vi "Team Editor and Schedule Creator.vi"(8 "Edit?":bool=TRUE, 11 "TeamData_and_Schedule IN":T2) -> (0 "LegacyTeamInfo":T1, 1 "RAW Schedule":string[][](array[string]), 2 "String Schedule":string[][](array[string]), 3 "TeamData_and_Schedule OUT":T2, 4 "MatchEqualizationString":string[][](array[string]), 5 "Cancelled?":bool=TRUE, 6 "MatchEqualizationInteger":i32[](array[numeric]))   [LabVIEW 2013]
uses:
  Team Data Array2.ctl
  TeamData_and_Schedule.ctl
  Legacy_Team_Info.ctl
  <vilib>/Utility/sysdir.llb/System Directory Type.ctl
  <vilib>/Utility/xml.llb/Write to XML File(string).vi
  <vilib>/Utility/xml.llb/Read From XML File(string).vi
panel:
  out "Team Number Schedule":i32[][](array[numeric])
  out "Match Array (indices)":i32[][](array[numeric])
  out "NextState":i32
  in  "Team Info":T3
  in  "Tab Control":T4(tab)
  out "String":string="NOTE:  You are not allowed to Add or Delete teams once you've started submitting scores for teams.  Doing so may drop scores, or assign scores to the wrong teams!\n\nOnce you've begun submitting scores, you are only allowed to edit the team information."
  in  "Load Team List Button":bool
  in  "Save Team List Button":bool
  in  "Number of Teams:":dbl
  in  "Cancel Button":bool
  in  "OK Button":bool
  in  "Edit Team Button":bool
  in  "Remove Team Button":bool
  in  "Add Team Button":bool
  in  "Competing Team List":i32(listbox)
  in  "Add Team Back Button":bool
  in  "Add Team Next Button":bool
  out "Add Team String":string="Add a Team\n\nEnter Team Information and press NEXT.  To cancel, press BACK.  You are required to provide a TEAM NUMBER greater than ZERO and a non-blank Team Name."
  in  "Team Number":dbl
  in  "Team Name":string
  in  "Remove Team Back Button":bool
  in  "Remove Team Next Button":bool
  out "Remove Team String":string="Remove a Team\n\nSelect Team to Remove and press NEXT.  To cancel, press BACK.  If you press NEXT, the selected team will be removed."
  in  "Team To Remove":u16(ring)
  in  "Edit Team Back Button":bool
  in  "Edit Team Next Button":bool
  out "Rename Team String":string="Rename a Team\n\nSelect a Team to be Renamed, then type in the NEW name of the team in the \"New Team Name\" field.  The New Team Name cannot be blank. Press NEXT to rename the team, or BACK to cancel."
  in  "Team to Edit":u16(ring) items=["10, Team One Oh"=0, "20, Twenty is Plenty"=1, "40, The Shorty Forty "=3, "42, The Ultimate Answer"=4, "50, Half Century Team"=5, "60, The Golden Years"=6, "70, One Plus LASA Robotics"=7, "80, Eighty is Greaty"=8, "90, Ten to a Century"=9, "100, Century Mark Team"=10]
  in  "New Team Name":string
  in  "New Team Number":dbl
  out "Error String":string
  in  "Error Back Button":bool
  in  "Back-To-Back Interval":dbl=1.0 min=0.0 max=8.0 step=1.0
  in  "Matches per Team":dbl=1.0 min=1.0 max=10.0 step=1.0
  in  "Number of Fields":dbl=1.0 min=1.0 max=2.0 step=1.0
  out "Create Schedule String":string="Create Schedule\n\nEnter the required information below.  \n\nNumber of Fields - Number of fields you have.  A field is composed of 4 quadrants that play simultaneously.\n\nMatches per Team - Number of matches each team is to be scheduled to play during the competition.\n\nBack-To-Back Interval - Minimum number of matches that can take place between when a team plays and when they have to play next."
  in  "CreateSched Back Button":bool
  in  "CreateSched Next Button":bool
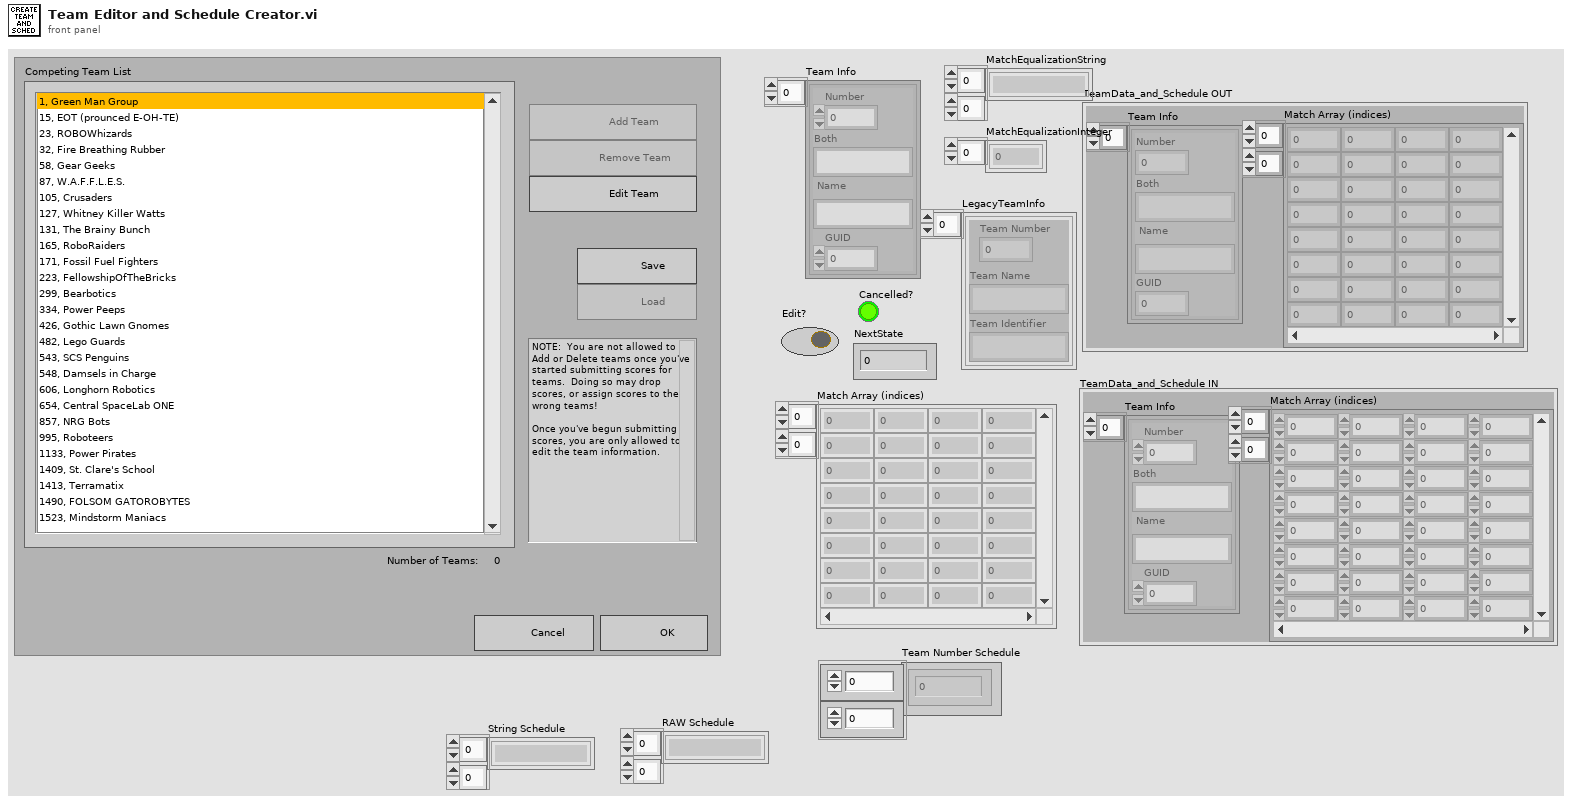
[diagram p1: front panel]
types:
  T1 = typedef "Legacy_Team_Info.ctl" = cluster{"Team Number":i32, "Team Name":string, "Team Identifier":string}[]
  T2 = typedef "TeamData_and_Schedule.ctl" = cluster{"Team Info":cluster{"Number":u16, "Both":string, "Name":string, "GUID":u16}[], "Match Array (indices)":i32[][]}
  T3 = typedef "Team Data Array2.ctl" = cluster{"Number":u16, "Both":string, "Name":string, "GUID":u16}[]
  T4 = enum32{"Main Page", "Add Team", "Remove Team", "Rename Team", "Errors", "Schedule"}
  T5 = enum8{"Enabled", "Disabled", "Disabled and Grayed Out"}
  T6 = cluster{"Number":u16, "Both":string, "Name":string, "GUID":u16}[]
  T7 = enum32{"Main Page", "Add Team", "Remove Team", "Rename Team", "Errors"}
  T8 = typedef "System Directory Type.ctl" = i32
  T9 = typedef "LVStringsAndValuesArrayTypeDef_U16.ctl" = cluster{"String":string, "Value":u16}[]
  T10 = cluster{"Team Number":i32, "Team Name":string, "Team Identifier":string}
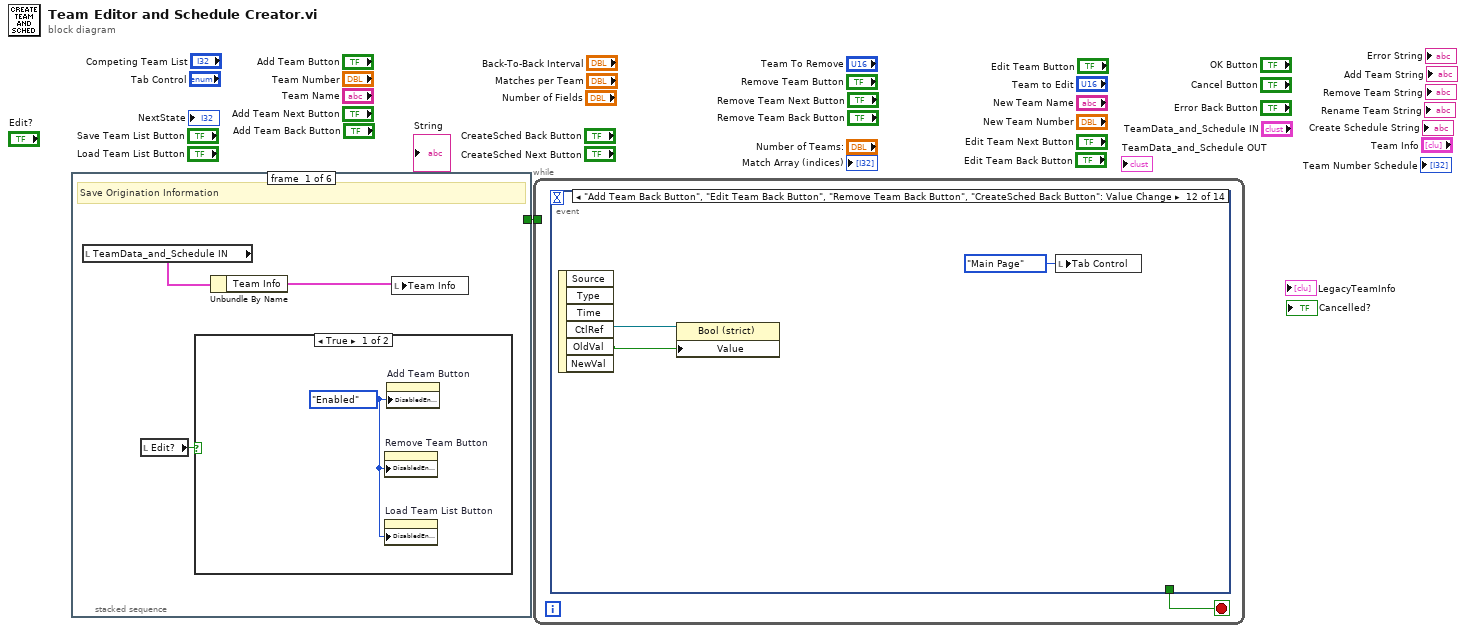
[diagram p0: block diagram]
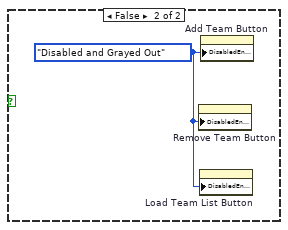
[diagram p2: hidden frame]
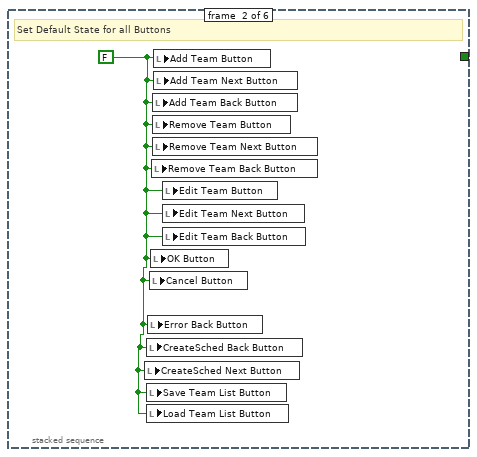
[diagram p3: hidden frame]
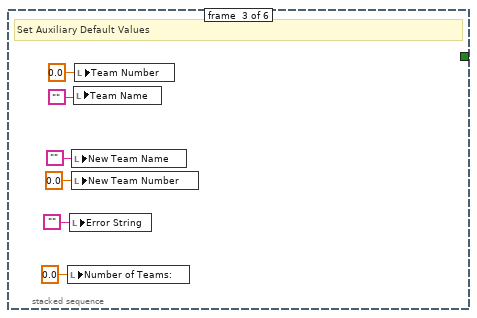
[diagram p4: hidden frame]
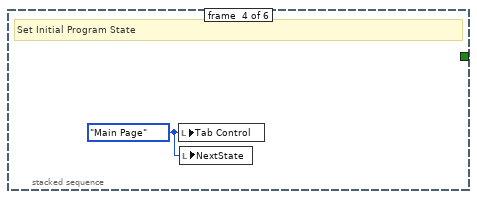
[diagram p5: hidden frame]
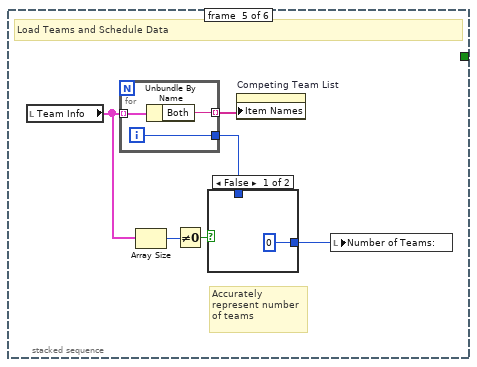
[diagram p6: hidden frame]
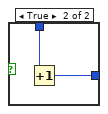
[diagram p7: hidden frame]
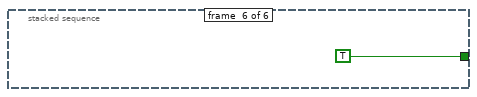
[diagram p8: hidden frame]
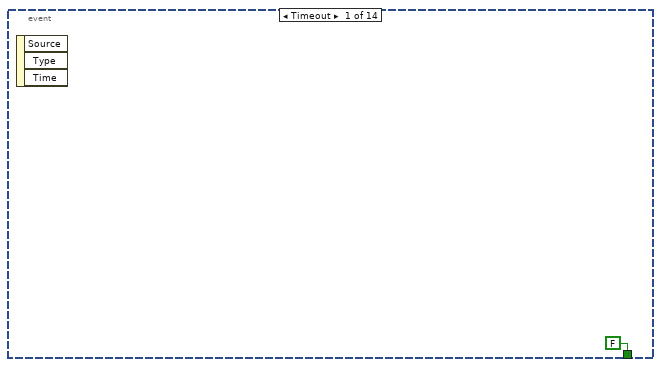
[diagram p9: hidden frame]
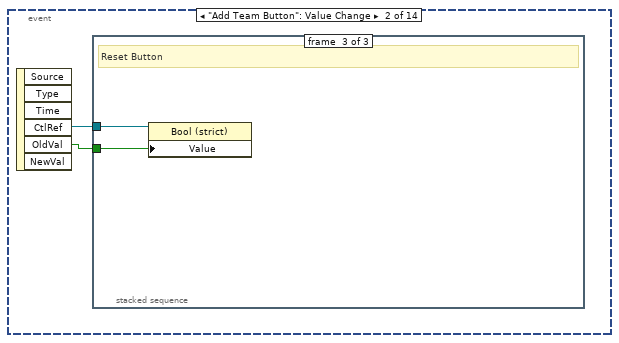
[diagram p10: hidden frame]
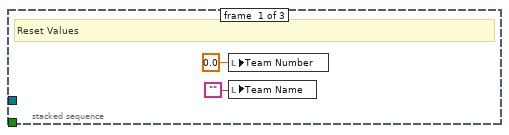
[diagram p11: hidden frame]
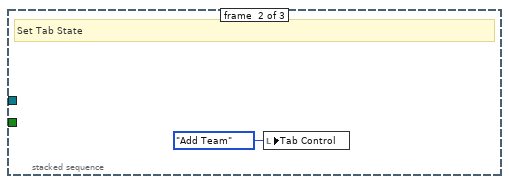
[diagram p12: hidden frame]
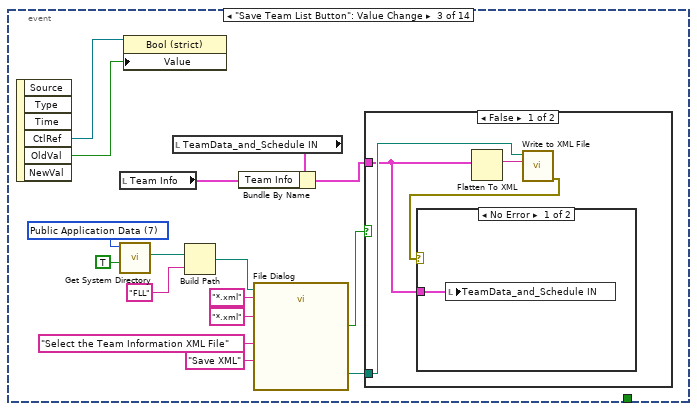
[diagram p13: hidden frame]
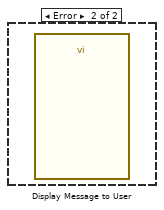
[diagram p14: hidden frame]
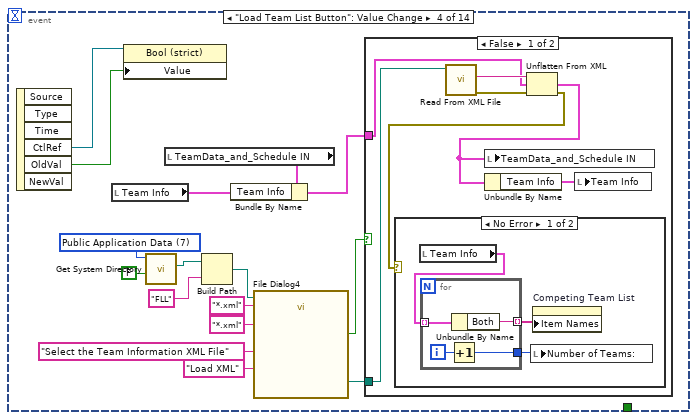
[diagram p16: hidden frame]
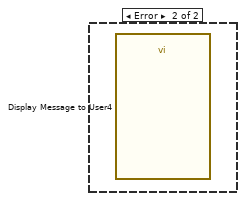
[diagram p17: hidden frame]
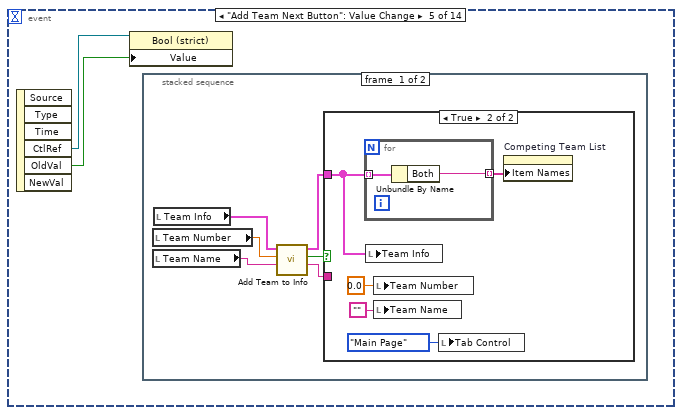
[diagram p19: hidden frame]
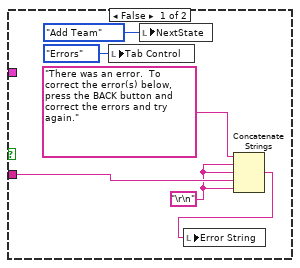
[diagram p20: hidden frame]
diagram:
  n1 = stacked-sequence {
    tunnel: [_ _ _ _ _ TRUE] -> w1
    frame #0 {
      # "Save Origination Information"
      n2 = local read "TeamData_and_Schedule IN"() -> (w4:T2)
      n3 = local read "Edit?"() -> (w2:bool)
      n4 = case shown="True" w2 {
        frame True {
          w5 = T5."Enabled" ("Disabled")
          n5 = property on="Remove Team Button" class="Bool (strict)"("DisabledEnum"=w5) -> ()  [unwired: 2 in, 2 out]
          n6 = property on="Load Team List Button" class="Bool (strict)"("DisabledEnum"=w5) -> ()  [unwired: 2 in, 2 out]
          n7 = property on="Add Team Button" class="Bool (strict)"("DisabledEnum"=w5) -> ()  [unwired: 2 in, 2 out]
        }
        frame False {
          w6 = T5."Disabled and Grayed Out" ("Disabled")
          n8 = property on="Remove Team Button" class="Bool (strict)"("DisabledEnum"=w6) -> ()  [unwired: 2 in, 2 out]
          n9 = property on="Load Team List Button" class="Bool (strict)"("DisabledEnum"=w6) -> ()  [unwired: 2 in, 2 out]
          n10 = property on="Add Team Button" class="Bool (strict)"("DisabledEnum"=w6) -> ()  [unwired: 2 in, 2 out]
        }
      }
      n11 = Unbundle By Name(w4) -> ("Team Info"=w3:T6)
      n12 = local write "Team Info"(w3) -> ()
    }
    frame #1 {
      w7 = FALSE
      # "Set Default State for all Buttons"
      n13 = local write "CreateSched Next Button"(w7) -> ()
      n14 = local write "CreateSched Back Button"(w7) -> ()
      n15 = local write "Save Team List Button"(w7) -> ()
      n16 = local write "Load Team List Button"(w7) -> ()
      n17 = local write "Error Back Button"(w7) -> ()
      n18 = local write "Cancel Button"(w7) -> ()
      n19 = local write "OK Button"(w7) -> ()
      n20 = local write "Remove Team Back Button"(w7) -> ()
      n21 = local write "Add Team Back Button"(w7) -> ()
      n22 = local write "Remove Team Button"(w7) -> ()
      n23 = local write "Remove Team Next Button"(w7) -> ()
      n24 = local write "Add Team Button"(w7) -> ()
      n25 = local write "Add Team Next Button"(w7) -> ()
      n26 = local write "Edit Team Button"(w7) -> ()
      n27 = local write "Edit Team Next Button"(w7) -> ()
      n28 = local write "Edit Team Back Button"(w7) -> ()
    }
    frame #2 {
      # "Set Auxiliary Default Values"
      n29 = local write "Number of Teams:"(0.0 ("Number of Teams:")) -> ()
      n30 = local write "Error String"("") -> ()
      n31 = local write "New Team Name"("") -> ()
      n32 = local write "New Team Number"(0.0 ("New Team Number")) -> ()
      n33 = local write "Team Name"("") -> ()
      n34 = local write "Team Number"(0.0 ("Team Number")) -> ()
    }
    frame #3 {
      w14 = T7."Main Page" ("Tab Control")
      # "Set Initial Program State"
      n35 = local write "Tab Control"(w14) -> ()
      n36 = local write "NextState"(w14) -> ()
    }
    frame #4 {
      # "Accurately \nrepresent number\nof teams"
      # "Load Teams and Schedule Data"
      n37 = local read "Team Info"() -> (w17:T3)
      n38 = for {
        tunnel: w17 -> [w26] mode=indexing
        tunnel: [w25] -> w20 mode=indexing
        tunnel: [w24] -> w19
        i -> [w24]
        n39 = Unbundle By Name(w26) -> ("Both"=w25:string)
      }
      n40 = Array Size(array=w17) -> (size(s)=w16:i32)
      n41 = Not Equal To 0?(x=w16) -> (x != 0?=w15:bool)
      n42 = case shown="False" w15 {
        tunnel: w19 -> [_ w23]
        tunnel: [0 w22] -> w18
        frame False {
        }
        frame True {
          n43 = Increment(x=w23) -> (x+1=w22:i32)
        }
      }
      n44 = property on="Competing Team List" class="LstBox (strict)"("Item Names"=w20) -> ()  [unwired: 2 in, 2 out]
      n45 = local write "Number of Teams:"(w18) -> ()
    }
    frame #5 {
    }
  }
  n46 = while {
    tunnel: w1 -> [_]
    stop <- w28 stop-if-true
    n47 = event shown="[11] \"Add Team Back Button\", \"Edit Team Back Button\", \"Remove Team Back Button\", \"CreateSched Back Button\": Value Change" {
      selector: _ -> [_ _ _ _ _ _ _ _ _ _ _ _ _ _]
      dyn-events: _ -> [_ _ _ _ _ _ _ _ _ _ _ _ _ _]
      timeout: _ -> [_ _ _ _ _ _ _ _ _ _ _ _ _ _]
      tunnel: [FALSE _ _ _ _ _ _ _ _ _ _ _ TRUE TRUE] -> w28
      event Timeout {
        n48 = event-data() -> ()  [unwired: 1 in, 3 out]
      }
      event "Add Team Button": Value Change {
        n49 = event-data() -> ("CtlRef"=w31:refnum<vi>, "OldVal"=w30:bool)  [unwired: 1 in, 4 out]
        n50 = stacked-sequence {
          tunnel: w31 -> [_ _ w36]
          tunnel: w30 -> [_ _ w35]
          frame #0 {
            # "Reset Values"
            n51 = local write "Team Number"(0.0 ("Team Number")) -> ()
            n52 = local write "Team Name"("") -> ()
          }
          frame #1 {
            # "Set Tab State"
            n53 = local write "Tab Control"(T7."Add Team" ("Tab Control")) -> ()
          }
          frame #2 {
            # "Reset Button"
            n54 = property class="Bool (strict)"(reference=w36, "Value"=w35) -> ()  [unwired: 1 in, 2 out]
          }
        }
      }
      event "Save Team List Button": Value Change {
        w44 = T8 7 items=["User Home"=0, "User Desktop"=1, "User Documents"=2, "User Application Data"=3, "User Preferences"=4, "User Temporary"=5, "Public Documents"=6, "Public Application Data"=7, "Public Preferences"=8, "Public Cache"=13, "System Core Libraries"=9, "System Installed Libraries"=10, "Application Files"=11, "Boot Volume Root"=12] ("system directory type")
        n55 = event-data() -> ("CtlRef"=w52:refnum<vi>, "OldVal"=w51:bool)  [unwired: 1 in, 4 out]
        n56 = local read "Team Info"() -> (w41:T3)
        n57 = call <vilib>:"Get System Directory.vi"("create directory if not found? (F)"=TRUE, "system directory type"=w44) -> ("system directory"=w39:path)  [unwired: 9 in]
        n58 = property class="Bool (strict)"(reference=w52, "Value"=w51) -> ()  [unwired: 1 in, 2 out]
        n59 = local read "TeamData_and_Schedule IN"() -> (w42:T2)
        n60 = Build Path(base path=w39, name or relative path="FLL") -> (appended path=w37:path)
        n61 = Bundle By Name(cluster=w42, "Team Info"=w41) -> (w40:T2)
        n62 = call "File Dialog"("start path"=w37, "prompt"="Select the Team Information XML File", "button label"="Save XML", "pattern (all files)"="*.xml", "pattern label"="*.xml") -> ("selected path"=w45:path, "cancelled"=w46:bool)  [unwired: 7 in, 2 out]
        n63 = case shown="False" w46 {
          tunnel: w45 -> [w55 _]
          tunnel: w40 -> [w53 _]
          frame False {
            n64 = Flatten To XML(anything=w53) -> (xml string=w56:string)
            n65 = call-poly <vilib>:"Write to XML File.vi"("XML Input"=w56, "XML File Path"=w55) -> ("error out"=w54:errorcluster)  [unwired: 7 in, 2 out]
            n66 = case shown="No Error" w54 {
              tunnel: w53 -> [w57 _]
              frame No Error {
                n67 = local write "TeamData_and_Schedule IN"(w57) -> ()
              }
              frame Error {
                n68 = call "Display Message to User"() -> ()  [unwired: 10 in, 2 out]
              }
            }
          }
          frame True {
          }
        }
      }
      event "Load Team List Button": Value Change {
        w65 = T8 7 items=["User Home"=0, "User Desktop"=1, "User Documents"=2, "User Application Data"=3, "User Preferences"=4, "User Temporary"=5, "Public Documents"=6, "Public Application Data"=7, "Public Preferences"=8, "Public Cache"=13, "System Core Libraries"=9, "System Installed Libraries"=10, "Application Files"=11, "Boot Volume Root"=12] ("system directory type")
        n69 = event-data() -> ("CtlRef"=w73:refnum<vi>, "OldVal"=w72:bool)  [unwired: 1 in, 4 out]
        n70 = local read "Team Info"() -> (w62:T3)
        n71 = property class="Bool (strict)"(reference=w73, "Value"=w72) -> ()  [unwired: 1 in, 2 out]
        n72 = call <vilib>:"Get System Directory.vi"("create directory if not found? (F)"=FALSE, "system directory type"=w65) -> ("system directory"=w60:path)  [unwired: 9 in]
        n73 = local read "TeamData_and_Schedule IN"() -> (w63:T2)
        n74 = Build Path(base path=w60, name or relative path="FLL") -> (appended path=w58:path)
        n75 = Bundle By Name(cluster=w63, "Team Info"=w62) -> (w61:T2)
        n76 = call "File Dialog4"("start path"=w58, "prompt"="Select the Team Information XML File", "button label"="Load XML", "pattern (all files)"="*.xml", "pattern label"="*.xml") -> ("selected path"=w66:path, "cancelled"=w67:bool)  [unwired: 7 in, 2 out]
        n77 = case shown="False" w67 {
          tunnel: w66 -> [w80 _]
          tunnel: w61 -> [w78 _]
          frame False {
            n78 = call-poly <vilib>:"Read From XML File.vi"("XML File Path"=w80) -> ("error out"=w76:errorcluster, "XML Elements"=w79:string)  [unwired: 8 in, 1 out]
            n79 = Unflatten From XML(xml string=w79, type=w78, error in (no error)=w76) -> (value=w74:T2, error out=w77:errorcluster)
            n80 = case shown="No Error" w77 {
              frame No Error {
                n81 = local read "Team Info"() -> (w83:T3)
                n82 = for {
                  tunnel: w83 -> [w87] mode=indexing
                  tunnel: [w86] -> w82 mode=indexing
                  tunnel: [w84] -> w81
                  i -> [w85]
                  n83 = Increment(x=w85) -> (x+1=w84:i32)
                  n84 = Unbundle By Name(w87) -> ("Both"=w86:string)
                }
                n85 = local write "Number of Teams:"(w81) -> ()
                n86 = property on="Competing Team List" class="LstBox (strict)"("Item Names"=w82) -> ()  [unwired: 2 in, 2 out]
              }
              frame Error {
                n87 = call "Display Message to User4"() -> ()  [unwired: 10 in, 2 out]
              }
            }
            n88 = local write "TeamData_and_Schedule IN"(w74) -> ()
            n89 = Unbundle By Name(w74) -> ("Team Info"=w75:T6)
            n90 = local write "Team Info"(w75) -> ()
          }
          frame True {
          }
        }
      }
      event "Add Team Next Button": Value Change {
        n91 = event-data() -> ("CtlRef"=w89:refnum<vi>, "OldVal"=w88:bool)  [unwired: 1 in, 4 out]
        n92 = property class="Bool (strict)"(reference=w89, "Value"=w88) -> ()  [unwired: 1 in, 2 out]
        n93 = stacked-sequence {
          frame #0 {
            n94 = local read "Team Number"() -> (w94:dbl)
            n95 = local read "Team Name"() -> (w95:string)
            n96 = local read "Team Info"() -> (w93:T3)
            n97 = call "Add Team to Info.vi"("Team Name"=w95, "Team Number"=w94, "Team Info in"=w93) -> ("Error String"=w90:string, "Team Added?"=w92:bool, "Team Info out"=w91:T3)  [unwired: 6 in]
            n98 = case shown="True" w92 {
              tunnel: w91 -> [_ w104]
              tunnel: w90 -> [w99 _]
              frame False {
                w98 = "\r\n"
                n99 = local write "Tab Control"(T7."Errors" ("Tab Control")) -> ()
                n100 = local write "NextState"(T7."Add Team" ("Tab Control")) -> ()
                n101 = Concatenate Strings("There was an error.  To correct the error(s) below, press the BACK button and correct the errors and try again.", w98, w98, w99, w98) -> (w97:string)
                n102 = local write "Error String"(w97) -> ()
              }
              frame True {
                n103 = for {
                  tunnel: w104 -> [w108] mode=indexing
                  tunnel: [w107] -> w106 mode=indexing
                  n104 = Unbundle By Name(w108) -> ("Both"=w107:string)
                }
                n105 = local write "Team Info"(w104) -> ()
                n106 = local write "Team Number"(0.0 ("Team Number")) -> ()
                n107 = local write "Team Name"("") -> ()
                n108 = local write "Tab Control"(T7."Main Page" ("Tab Control")) -> ()
                n109 = property on="Competing Team List" class="LstBox (strict)"("Item Names"=w106) -> ()  [unwired: 2 in, 2 out]
              }
            }
          }
          frame #1 {
            n110 = property on="Competing Team List" class="LstBox (strict)"() -> ("Item Names"=w110:string[])  [unwired: 2 in, 2 out]
            n111 = Array Size(array=w110) -> (size(s)=w109:i32)
            n112 = local write "Number of Teams:"(w109) -> ()
          }
        }
      }
      event "Edit Team Next Button": Value Change {
        n113 = event-data() -> ("CtlRef"=w112:refnum<vi>, "OldVal"=w111:bool)  [unwired: 1 in, 4 out]
        n114 = stacked-sequence {
          frame #0 {
            n115 = local read "New Team Number"() -> (w118:dbl)
            n116 = local read "New Team Name"() -> (w119:string)
            n117 = local read "Team to Edit"() -> (w113:u16)
            n118 = local read "Team Info"() -> (w117:T3)
            n119 = call "Edit Team in Info.vi"("Team GUID"=w113, "New Team Name"=w119, "New Team Number"=w118, "Team Info in"=w117) -> ("Error String"=w114:string, "Team Edited?"=w116:bool, "Team Info out"=w115:T3)  [unwired: 5 in]
            n120 = case shown="False" w116 {
              tunnel: w115 -> [_ w128]
              tunnel: w114 -> [w123 _]
              frame False {
                w122 = "\r\n"
                n121 = local write "Tab Control"(T7."Errors" ("Tab Control")) -> ()
                n122 = local write "NextState"(T7."Rename Team" ("Tab Control")) -> ()
                n123 = Concatenate Strings("There was an error.  To correct the error(s) below, press the BACK button and correct the errors and try again.", w122, w122, w123, w122) -> (w121:string)
                n124 = local write "Error String"(w121) -> ()
              }
              frame True {
                n125 = for {
                  tunnel: w128 -> [w132] mode=indexing
                  tunnel: [w131] -> w130 mode=indexing
                  n126 = Unbundle By Name(w132) -> ("Both"=w131:string)
                }
                n127 = local write "Team Info"(w128) -> ()
                n128 = local write "New Team Number"(0.0 ("Team Number")) -> ()
                n129 = local write "New Team Name"("") -> ()
                n130 = local write "Tab Control"(T7."Main Page" ("Tab Control")) -> ()
                n131 = property on="Competing Team List" class="LstBox (strict)"("Item Names"=w130) -> ()  [unwired: 2 in, 2 out]
              }
            }
          }
          frame #1 {
            n132 = property on="Competing Team List" class="LstBox (strict)"() -> ("Item Names"=w134:string[])  [unwired: 2 in, 2 out]
            n133 = Array Size(array=w134) -> (size(s)=w133:i32)
            n134 = local write "Number of Teams:"(w133) -> ()
          }
        }
        n135 = property class="Bool (strict)"(reference=w112, "Value"=w111) -> ()  [unwired: 1 in, 2 out]
      }
      event "Error Back Button": Value Change {
        n136 = event-data() -> ("CtlRef"=w136:refnum<vi>, "OldVal"=w135:bool)  [unwired: 1 in, 4 out]
        n137 = property class="Bool (strict)"(reference=w136, "Value"=w135) -> ()  [unwired: 1 in, 2 out]
        n138 = local read "NextState"() -> (w137:i32)
        n139 = local write "Tab Control"(w137) -> ()
      }
      event "Remove Team Button": Value Change {
        n140 = event-data() -> ("CtlRef"=w139:refnum<vi>, "OldVal"=w138:bool)  [unwired: 1 in, 4 out]
        n141 = stacked-sequence {
          tunnel: w139 -> [_ _ w155]
          tunnel: w138 -> [_ _ w154]
          frame #0 {
            # "Reset Values"
            n142 = stacked-sequence {
              frame #0 {
                n143 = local read "Team Info"() -> (w141:T3)
                n144 = for {
                  tunnel: w141 -> [w145] mode=indexing
                  tunnel: [w142] -> w140 mode=indexing
                  n145 = Unbundle By Name(w145) -> ("Both"=w143:string, "GUID"=w144:u16)
                  n146 = Bundle("Both"=w143, "GUID"=w144) -> (w142:cluster{"Both":string, "GUID":u16})  [unwired: 1 in]
                }
                n147 = property on="Team To Remove" class="Ring (strict)"("StringsAndValues[]"=w140) -> ()  [unwired: 2 in, 2 out]
              }
              frame #1 {
                n148 = local read "Competing Team List"() -> (w149:i32)
                n149 = property on="Team To Remove" class="Ring (strict)"() -> ("StringsAndValues[]"=w152:T9)  [unwired: 2 in, 2 out]
                n150 = In Range and Coerce(upper limit=1000, x=w149, lower limit=0) -> (coerced(x)=w148:i32)  [unwired: 1 out]
                n151 = Index Array(array=w152, index=w148) -> (element=w151:cluster{"String":string, "Value":u16})
                n152 = Unbundle By Name(w151) -> ("Value"=w150:u16)
                n153 = property on="Team To Remove" class="Ring (strict)"("Value"=w150) -> ()  [unwired: 2 in, 2 out]
              }
            }
          }
          frame #1 {
            # "Set Tab State"
            n154 = local write "Tab Control"(T7."Remove Team" ("Tab Control")) -> ()
          }
          frame #2 {
            # "Reset Button"
            n155 = property class="Bool (strict)"(reference=w155, "Value"=w154) -> ()  [unwired: 1 in, 2 out]
          }
        }
      }
      event "Remove Team Next Button": Value Change {
        n156 = event-data() -> ("CtlRef"=w156:refnum<vi>, "OldVal"=w157:bool)  [unwired: 1 in, 4 out]
        n157 = property class="Bool (strict)"(reference=w156, "Value"=w157) -> ()  [unwired: 1 in, 2 out]
        n158 = stacked-sequence {
          frame #0 {
            n159 = local read "Team Info"() -> (w160:T3)
            n160 = property on="Team To Remove" class="Ring (strict)"() -> ("Value"=w159:u16)  [unwired: 2 in, 2 out]
            n161 = for {
              tunnel: w160 -> [w163] mode=indexing
              tunnel: w159 -> [w164]
              tunnel: [w163] -> w158 mode=indexing if=w161
              n162 = Unbundle By Name(w163) -> ("GUID"=w165:u16)
              n163 = Equal?(x=w165, y=w164) -> (x = y?=w162:bool)
              n164 = Not(x=w162) -> (.not. x?=w161:bool)
            }
            n165 = local write "Team Info"(w158) -> ()
          }
          frame #1 {
            n166 = local read "Team Info"() -> (w166:T3)
            n167 = for {
              tunnel: w166 -> [w169] mode=indexing
              tunnel: [w168] -> w167 mode=indexing
              n168 = Unbundle By Name(w169) -> ("Both"=w168:string)
            }
            n169 = property on="Competing Team List" class="LstBox (strict)"("Item Names"=w167) -> ()  [unwired: 2 in, 2 out]
          }
          frame #2 {
            n170 = local write "Tab Control"(T7."Main Page" ("Tab Control")) -> ()
          }
          frame #3 {
            n171 = property on="Competing Team List" class="LstBox (strict)"() -> ("Item Names"=w172:string[])  [unwired: 2 in, 2 out]
            n172 = Array Size(array=w172) -> (size(s)=w171:i32)
            n173 = local write "Number of Teams:"(w171) -> ()
          }
        }
      }
      event "Edit Team Button": Value Change {
        n174 = event-data() -> ("CtlRef"=w174:refnum<vi>, "OldVal"=w173:bool)  [unwired: 1 in, 4 out]
        n175 = stacked-sequence {
          tunnel: w174 -> [_ _ w206]
          tunnel: w173 -> [_ _ w205]
          frame #0 {
            # "Reset Values"
            n176 = stacked-sequence {
              frame #0 {
                n177 = local read "Team Info"() -> (w177:T3)
                n178 = for {
                  tunnel: w177 -> [w181] mode=indexing
                  tunnel: [w178] -> w176 mode=indexing
                  n179 = Unbundle By Name(w181) -> ("Both"=w179:string, "GUID"=w180:u16)
                  n180 = Bundle("Both"=w179, "GUID"=w180) -> (w178:cluster{"Both":string, "GUID":u16})  [unwired: 1 in]
                }
                n181 = property on="Team to Edit" class="Ring (strict)"("StringsAndValues[]"=w176) -> ()  [unwired: 2 in, 2 out]
              }
              frame #1 {
                n182 = local read "Competing Team List"() -> (w185:i32)
                n183 = property on="Team to Edit" class="Ring (strict)"() -> ("StringsAndValues[]"=w187:T9)  [unwired: 2 in, 2 out]
                n184 = In Range and Coerce(upper limit=1000, x=w185, lower limit=0) -> (coerced(x)=w182:i32)  [unwired: 1 out]
                n185 = Index Array(array=w187, index=w182) -> (element=w188:cluster{"String":string, "Value":u16})
                n186 = Unbundle By Name(w188) -> ("Value"=w186:u16)
                n187 = property on="Team to Edit" class="Ring (strict)"("Value"=w186) -> ()  [unwired: 2 in, 2 out]
              }
              frame #2 {
                n188 = local read "Team Info"() -> (w192:T3)
                n189 = property on="Team to Edit" class="Ring (strict)"() -> ("Value"=w193:u16)  [unwired: 2 in, 2 out]
                n190 = for {
                  tunnel: w193 -> [w201]
                  tunnel: w192 -> [w203] mode=indexing
                  tunnel: [w200] -> w190
                  tunnel: [w199] -> w189
                  tunnel: [w198] -> w191
                  stop <- w198 stop-if-true
                  n191 = Unbundle By Name(w203) -> ("GUID"=w202:u16, "Name"=w200:string, "Number"=w199:u16)
                  n192 = Equal?(x=w201, y=w202) -> (x = y?=w198:bool)
                }
                n193 = case shown="False" w191 {
                  tunnel: w190 -> [w195 _]
                  tunnel: w189 -> [w194 _]
                  frame True {
                    n194 = local write "New Team Name"(w195) -> ()
                    n195 = local write "New Team Number"(w194) -> ()
                  }
                  frame False {
                    n196 = local write "New Team Number"(0.0 ("New Team Number")) -> ()
                    n197 = local write "New Team Name"("<ERROR>") -> ()
                  }
                }
              }
            }
            n198 = local write "New Team Name"("") -> ()
          }
          frame #1 {
            # "Set Tab State"
            n199 = local write "Tab Control"(T7."Rename Team" ("Tab Control")) -> ()
          }
          frame #2 {
            # "Reset Button"
            n200 = property class="Bool (strict)"(reference=w206, "Value"=w205) -> ()  [unwired: 1 in, 2 out]
          }
        }
      }
      event "Team to Edit": Value Change {
        n201 = event-data() -> ()  [unwired: 1 in, 6 out]
        n202 = local read "Team Info"() -> (w210:T3)
        n203 = property on="Team to Edit" class="Ring (strict)"() -> ("Value"=w211:u16)  [unwired: 2 in, 2 out]
        n204 = for {
          tunnel: w211 -> [w219]
          tunnel: w210 -> [w221] mode=indexing
          tunnel: [w218] -> w208
          tunnel: [w217] -> w207
          tunnel: [w216] -> w209
          stop <- w216 stop-if-true
          n205 = Unbundle By Name(w221) -> ("GUID"=w220:u16, "Name"=w218:string, "Number"=w217:u16)
          n206 = Equal?(x=w219, y=w220) -> (x = y?=w216:bool)
        }
        n207 = case shown="False" w209 {
          tunnel: w208 -> [w213 _]
          tunnel: w207 -> [w212 _]
          frame True {
            n208 = local write "New Team Name"(w213) -> ()
            n209 = local write "New Team Number"(w212) -> ()
          }
          frame False {
            n210 = local write "New Team Number"(0.0 ("New Team Number")) -> ()
            n211 = local write "New Team Name"("<ERROR>") -> ()
          }
        }
      }
      event "Add Team Back Button", "Edit Team Back Button", "Remove Team Back Button", "CreateSched Back Button": Value Change {
        n212 = event-data() -> ("CtlRef"=w222:refnum<vi>, "OldVal"=w223:bool)  [unwired: 1 in, 4 out]
        n213 = property class="Bool (strict)"(reference=w222, "Value"=w223) -> ()  [unwired: 1 in, 2 out]
        n214 = local write "Tab Control"(T7."Main Page" ("Tab Control")) -> ()
      }
      event "OK Button": Value Change {
        n215 = event-data() -> ()  [unwired: 1 in, 6 out]
        n216 = local read "Match Array (indices)"() -> (w234:i32[][])
        n217 = local read "Team Info"() -> (w232:T3)
        n218 = local read "TeamData_and_Schedule OUT"() -> (w235:T2)
        n219 = local read "LegacyTeamInfo"() -> (w231:T1)
        n220 = Bundle By Name(cluster=w235, "Team Info"=w232, "Match Array (indices)"=w234) -> (w236:T2)
        n221 = call "Translate Schedule to Teams.vi"("Match Array (indices)"=w234, "Team Info Out"=w232) -> ("String Schedule"=→"String Schedule":string[][], "RAW Schedule"=w229:string[][])  [unwired: 9 in, 3 out]
        "RAW Schedule" <- w229
        n222 = call "FindMatchEqualizationPoints.vi"("RawSchedule"=w229) -> ("Array 2"=→"MatchEqualizationString":string[][], "Array"=→"MatchEqualizationInteger":i32[])  [unwired: 9 in]
        n223 = Index Array(array=w231) -> (element=w230:T10)  [unwired: 1 in]
        n224 = for {
          tunnel: w232 -> [w243] mode=indexing
          tunnel: w230 -> [w242]
          tunnel: [w238] -> w225 mode=indexing
          n225 = Unbundle By Name(w243) -> ("Number"=w241:u16, "Name"=w240:string, "Both"=w239:string)
          n226 = Bundle By Name(cluster=w242, "Team Number"=w241, "Team Name"=w240, "Team Identifier"=w239) -> (w238:T10)
        }
        n227 = local write "TeamData_and_Schedule OUT"(w236) -> ()
        n228 = local write "LegacyTeamInfo"(w225) -> ()
        n229 = local write "Cancelled?"(FALSE ("Cancelled?")) -> ()
      }
      event "Cancel Button": Value Change {
        n230 = event-data() -> ()  [unwired: 1 in, 6 out]
        n231 = local read "TeamData_and_Schedule IN"() -> (w245:T2)
        n232 = local write "TeamData_and_Schedule OUT"(w245) -> ()
        n233 = local write "Cancelled?"(TRUE) -> ()
      }
    }
  }
